vi "scantest.vi"() -> ()   [LabVIEW 2019]
uses:
  <vilib>/rvi/interface/nirviMethod/nirviMethod.xnode
  <vilib>/rvi/interface/nirviMethod/StockFPGA_InlinedMethodWaitForSingleIRQ.vi
  <vilib>/FPGAPlugInAG/Dynamic/niLvFpga_WaitOnIrq_Dynamic.vi
  <vilib>/rvi/interface/nirviReadWriteControl/nirviReadWriteControl.xnode
  <vilib>/FPGAPlugInAG/Dynamic/niLvFpga_AcknowledgeIrq_Dynamic.vi
  <vilib>/rvi/interface/nirviOpenFPGA/nirviOpenFPGA.xnode
  <vilib>/rvi/interface/nirviCloseFPGA/nirviCloseFPGA.xnode
  C:/Program Files (x86)/National Instruments/LabVIEW 2019/examples/CompactRIO/Module Specific/NI 9219/NI 9219 Scaling Utility/NI 9219 Scaling Support Files.llb/NI 9219 Convert Calibrated FXP to Thermocouple.vi
  C:/Program Files (x86)/National Instruments/LabVIEW 2019/examples/CompactRIO/Shared/cRIO Convert Thermocouple Readings.llb/Thermocouple Type.ctl
  FPGA Bitfiles/sbrio-9642sauna_FPGATarget2_Sauna9642FPGAMai_7whTey65SL0.lvbitx
  Sauna_9642_FPGA_Main.vi
  NiFpgaLv.dll
  <vilib>/Utility/error.llb/Error Cluster From Error Code.vi
  <vilib>/rvi/interface/Simulation/niFpgaSimulationCallBeginRW.vi
  <vilib>/rvi/errors/niLvFpgaAdjustHostInterfaceError.vi
  <vilib>/FPGAPlugInAG/Dynamic/niLvFpga_Close_Dynamic.vi
  <vilib>/FPGAPlugInAG/sbRIO-9642/niLvFpga_Open_sbRIO-9642.vi
  <vilib>/rvi/interface/common/dynamic/niFpgaDynamicAddResources.vi
panel:
  out "Data":T1
  in  "stop":bool
  out "Analog Data":T2(graph)
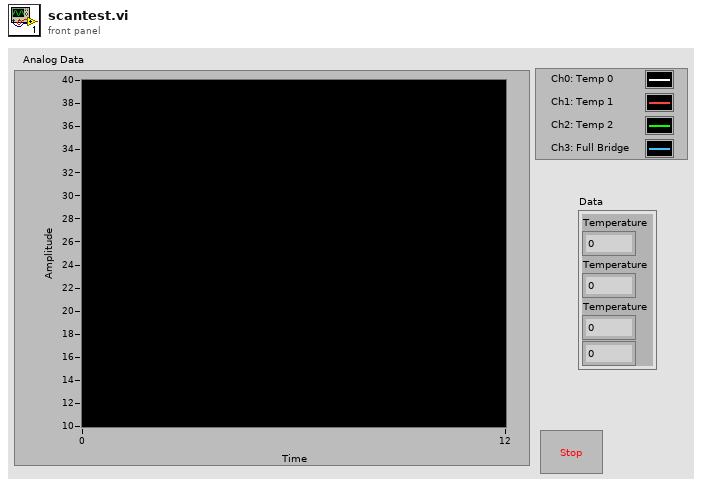
[diagram p1: front panel]
types:
  T1 = cluster{"Temperature":dbl, "Temperature":dbl, "Temperature":dbl, dbl}
  T2 = cluster{"Voltage (V)":dbl, "Temperature":dbl, "Temperature":dbl, "Strain (mV/V)":dbl}
  T3 = typedef "Thermocouple Type.ctl" = u16
  T4 = cluster{"TC0":fxp<+/-,32,-1>, "CJC0":fxp<+/-,32,-1>, "Switch":bool, "RTD":fxp<+,32,14>, "Bridge":fxp<+/-,32,-1>}
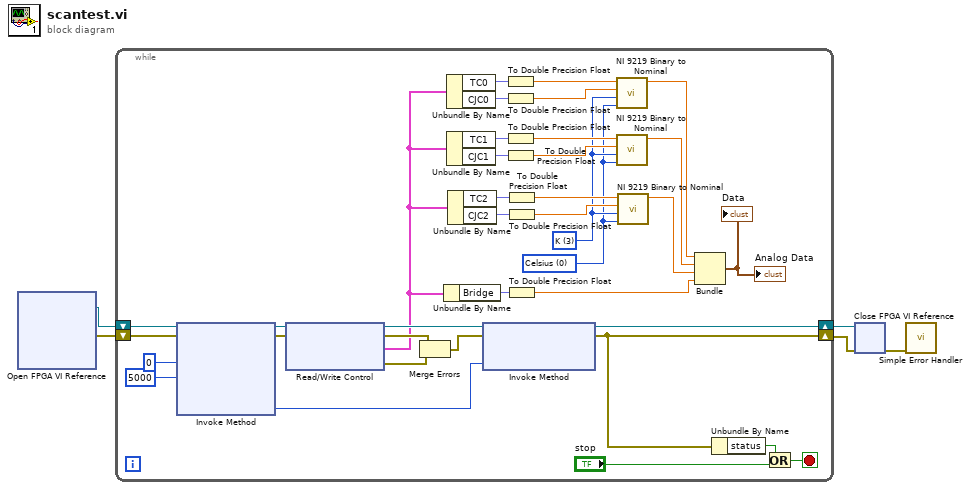
[diagram p0: block diagram]
diagram:
  n1 = xnode "Open FPGA VI Reference"() -> ("FPGA VI Reference Out"=w2:refnum<k20>, "error out"=w1:errorcluster)  [unwired: 2 in]
  n2 = while {
    shift-right: [w36] -> w5
    shift-left: w2 -> [w42]
    shift-right: [w33] -> w4
    shift-left: w1 -> [w41]
    stop <- w34 stop-if-true
    w7 = T3 3 items=["B", "E", "J", "K", "R", "S", "T", "N"] ("CH1 ThermocoupleType")
    w6 = u16 0 items=["Celsius", "Fahrenheit", "Kelvin", "Rankine"] ("CH1 Temperature Units")
    n3 = xnode "Invoke Method"("FPGA VI Reference In"=w42, "error in"=w41, "IRQ Number(s)"=0, "Timeout (ms)"=5000 ("timeout (ms)(-1 for no timeout)")) -> ("FPGA VI Reference Out"=w38:refnum<k20>, "error out"=w37:errorcluster, "IRQ(s) Asserted"=w35:i32)  [unwired: 1 out]
    n4 = xnode "Read/Write Control"("FPGA VI Reference In"=w38, "error in"=w37) -> ("FPGA VI Reference Out"=w30:refnum<k20>, "error out"=w27:errorcluster, "9219 Output"=w11:T4, "FPGA Error Out"=w26:errorcluster)
    n5 = Merge Errors(w27, w26) -> (w25:errorcluster)
    n6 = Unbundle By Name(w11) -> ("Bridge"=w24:fxp<+/-,32,-1>)
    n7 = Unbundle By Name(w11) -> ("TC0"=w15:fxp<+/-,32,-1>, "CJC0"=w14:fxp<+/-,32,-1>)
    n8 = Unbundle By Name(w11) -> ("TC1"=w16:fxp<+/-,32,-1>, "CJC1"=w17:fxp<+/-,32,-1>)
    n9 = Unbundle By Name(w11) -> ("TC2"=w28:fxp<+/-,32,-1>, "CJC2"=w22:fxp<+/-,32,-1>)
    n10 = xnode "Invoke Method"("FPGA VI Reference In"=w30, "error in"=w25, "IRQ Number(s)"=w35) -> ("FPGA VI Reference Out"=w36:refnum<k20>, "error out"=w33:errorcluster)
    n11 = To Double Precision Float(number=w15) -> (double precision float=w13:dbl)
    n12 = To Double Precision Float(number=w14) -> (double precision float=w12:dbl)
    n13 = To Double Precision Float(number=w16) -> (double precision float=w18:dbl)
    n14 = To Double Precision Float(number=w17) -> (double precision float=w19:dbl)
    n15 = To Double Precision Float(number=w28) -> (double precision float=w21:dbl)
    n16 = To Double Precision Float(number=w22) -> (double precision float=w20:dbl)
    n17 = To Double Precision Float(number=w24) -> (double precision float=w23:dbl)
    n18 = call-poly "NI 9219 Binary to Nominal.vi"("Temperature Units (C)"=w6, "ThermocoupleType"=w7, "CJC"=w12, "ADC Value"=w13) -> ("Temperature"=w10:dbl)  [unwired: 7 out]
    n19 = call-poly "NI 9219 Binary to Nominal.vi"("Temperature Units (C)"=w6, "ThermocoupleType"=w7, "CJC"=w19, "ADC Value"=w18) -> ("Temperature"=w9:dbl)  [unwired: 7 out]
    n20 = call-poly "NI 9219 Binary to Nominal.vi"("Temperature Units (C)"=w6, "ThermocoupleType"=w7, "CJC"=w20, "ADC Value"=w21) -> ("Temperature"=w29:dbl)  [unwired: 7 out]
    n21 = Bundle("Temperature"=w10, "Temperature"=w9, "Temperature"=w29, w23) -> (→"Analog Data" →"Data":T1)  [unwired: 1 out]
    n22 = Unbundle By Name(w33) -> ("status"=w32:bool)
    n23 = Or(x=w32, y="stop") -> (x .or. y?=w34:bool)
  }
  n24 = xnode "Close FPGA VI Reference"("FPGA VI Reference In"=w5, "error in"=w4) -> ("error out"=w3:errorcluster)
  n25 = call <vilib>:"Simple Error Handler.vi"("error in (no error)"=w3) -> ()  [unwired: 1 in, 8 out]
